vi "ReadFloats.vi"(1 "VISA resource name in":refnum<visa-resource-name>, 4 "Enable":bool, 5 "error in":errorcluster) -> (13 "status":bool, 14 "VISA resource name out":refnum<visa-resource-name>, 15 "error out":errorcluster, 16 "Float1":sgl, 17 "Float2":sgl, 18 "Float3":sgl, 19 "Float4":sgl)   [LabVIEW 2009]
panel:
  out "read buffer":string
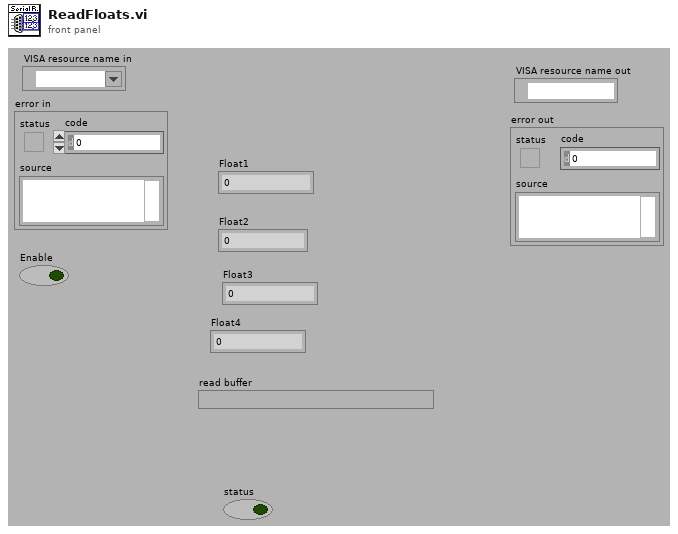
[diagram p1: front panel]
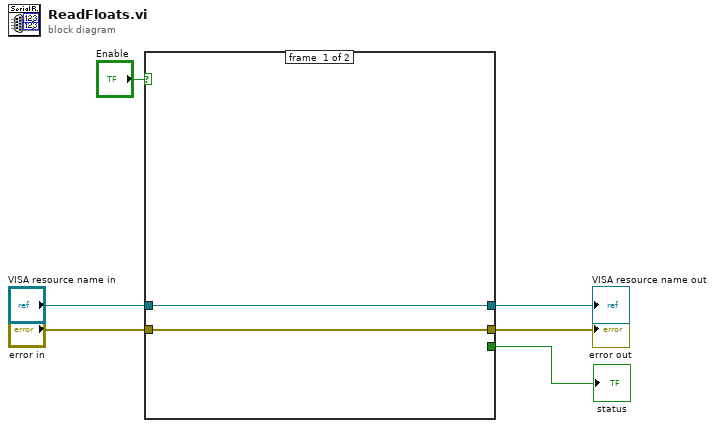
[diagram p0: block diagram]
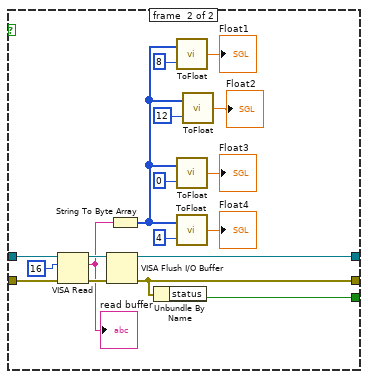
[diagram p2: hidden frame]
diagram:
  n1 = case shown="True" "Enable" {
    tunnel: [w7 w26] -> w1
    tunnel: [_ w9] -> w2
    tunnel: "error in" -> [w7 w23]
    tunnel: "VISA resource name in" -> [w8 w22]
    tunnel: [w8 w20] -> w6
    frame #0 {
    }
    frame #1 {
      n2 = VISA Read(VISA resource name=w22, byte count=u32 16 ("baud rate (9600)"), error in (no error)=w23) -> (VISA resource name out=w25:refnum<visa-resource-name>, read buffer=w19:string, error out=w24:errorcluster)  [unwired: 1 out]
      "read buffer" <- w19
      n3 = VISA Flush I/O Buffer(VISA resource name=w25, error in (no error)=w24) -> (VISA resource name out=w20:refnum<visa-resource-name>, error out=w26:errorcluster)  [unwired: 1 in]
      n4 = String To Byte Array(string=w19) -> (unsigned byte array=w10:u8[])
      n5 = Unbundle By Name(w26) -> ("status"=w9:bool)
      n6 = call "ToFloat.vi"("index"=8, "array"=w10) -> ("sp float"=→"Float1":sgl)
      n7 = call "ToFloat.vi"("index"=0, "array"=w10) -> ("sp float"=→"Float3":sgl)
      n8 = call "ToFloat.vi"("index"=4, "array"=w10) -> ("sp float"=→"Float4":sgl)
      n9 = call "ToFloat.vi"("index"=12, "array"=w10) -> ("sp float"=→"Float2":sgl)
    }
  }
  "VISA resource name out" <- w6
  "status" <- w2
  "error out" <- w1
